vi "LVDimInterface.dim_enable_security.vi"(2 "allowedNodes":string[](array[string]), 5 "error in (no error)":errorcluster) -> (19 "error out":errorcluster)   [LabVIEW 2012, in "LVDimInterface.lvlib"]
doc: "Enables security features for DIM. Only services received from the nodes that are specified here are allowed to access.\n\nHistory: 10-MAR-2006, Dietrich Beck\n\nCopyright (C)\nGesellschaft für Schwerionenforschung, GSI\nPlanckstr. 1\n64291 Darmstadt\nGermany\n\nContact: D.Beck@gsi.de \n\nThis program is free software; you can redistribute it and/or modify it under the terms of the \nGNU General Public License as published by the Free Software Foundation; either version 2 of the license, or (at your option) any later version.\n\nThis program is distributed in the hope that it will be useful, but WITHOUT ANY WARRANTY; without even the implied warranty of MERCHANTABILITY or FITNESS FOR A PARTICULAR PURPOSE. See the GNU General License for more details (http://www.gnu.org).\n\nGesellschaft für Schwerionenforschung, GSI\nPlanckstr. 1, 64291 Darmstadt, Germany\nFor all questions and ideas contact D. Beck.\nLast update: 16-DEC-2005"
uses:
  LVDimInterface.lvlib
  bin/libDimWrapper.dll
  bin/libDimWrapper.so
  bin/libDimWrapperSPL.dll
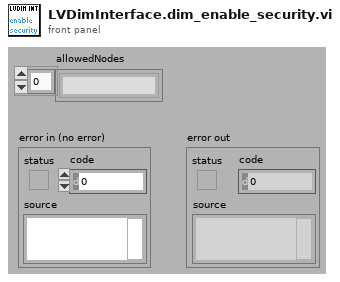
[diagram p1: front panel]
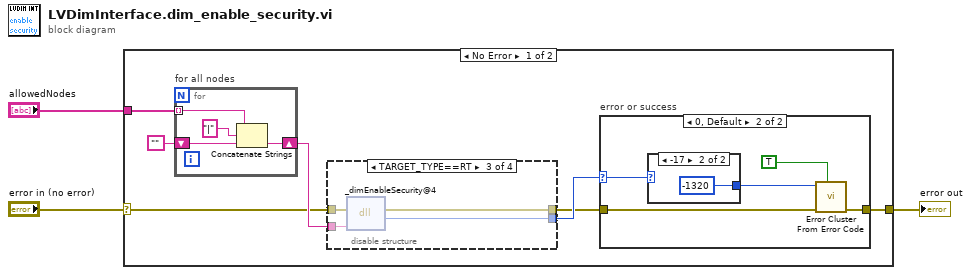
[diagram p0: block diagram]
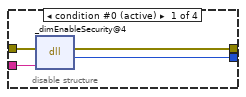
[diagram p2: hidden frame]
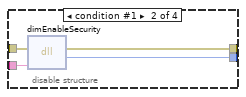
[diagram p3: hidden frame]
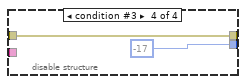
[diagram p4: hidden frame]
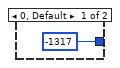
[diagram p6: hidden frame]
diagram:
  n1 = case shown="No Error" "error in (no error)" {
    selector: "error in (no error)" -> [w5 w37]
    tunnel: [w10 w37] -> w2
    tunnel: "allowedNodes" -> [w6 _]
    frame No Error {
      n2 = for "for all nodes" {
        shift-right: [w27] -> w7
        shift-left: "" ("Empty String Constant") -> [w28]
        tunnel: w6 -> [w26] mode=indexing
        n3 = Concatenate Strings(w26, "|" ("string"), w28) -> (w27:string)
      }
      n4 = disable-structure "Conditional Disable Structure" shown="TARGET_TYPE==RT" {
        disable-tunnel: [w14 w18 w22 -17 ("success")] -> w9
        disable-tunnel: w7 -> [w13 w17 w21 _]
        disable-tunnel: w5 -> [w12 w15 w20 w23]
        disable-tunnel: [w11 w16 w19 w23] -> w4
        frame condition #0 (active) {
          n5 = dll-call lib="D:/DIMLVEvent LV2012/bin/libDimWrapper.dll" fn="_dimEnableSecurity@4" label="dimEnableSecurity"(error in=w12, "allowedNodes"=w13) -> (error out=w11:errorcluster, "success"=w14:i32)  [unwired: 3 in, 1 out]
        }
        frame condition #1 {
          n6 = dll-call lib="D:/DIMLVEvent LV2012/bin/libDimWrapper.so" fn="dimEnableSecurity"(error in=w15, "allowedNodes"=w17) -> (error out=w16:errorcluster, "success"=w18:i32)  [unwired: 3 in, 1 out]
        }
        frame condition #2 {
          n7 = dll-call lib="D:/DIMLVEvent LV2012/bin/libDimWrapperSPL.dll" fn="_dimEnableSecurity@4" label="libDimWrapper.so:dimEnableSecurity"(error in=w20, "allowedNodes"=w21) -> (error out=w19:errorcluster, "success"=w22:i32)  [unwired: 3 in, 1 out]
        }
        frame condition #3 {
        }
      }
      n8 = case "error or success" shown="0, Default" w9 {
        selector: w9 -> [_ w34]
        tunnel: w4 -> [w29 w33]
        tunnel: [w29 w32] -> w10
        frame 1 {
        }
        frame 0, Default {
          n9 = case shown="-17" w34 {
            tunnel: [-1317 ("code") -1320 ("code")] -> w31
            frame 0, Default {
            }
            frame -17 {
            }
          }
          n10 = call <vilib>:"Error Cluster From Error Code.vi"("show call chain? (False)"=TRUE ("status"), "error in (no error)"=w33, "error code (0)"=w31) -> ("error out"=w32:errorcluster)  [unwired: 6 in]
        }
      }
    }
    frame Error {
    }
  }
  "error out" <- w2
